vi "Read Analogue.vi"(8 "error in (no error)":errorcluster, 11 "Keysight 6700C in":refnum<class "Keysight 6700C.lvclass">) -> (0 "error out":errorcluster, 2 "Waveforms":waveform(dbl)[](array[waveform]), 3 "Keysight 6700C out":refnum<class "Keysight 6700C.lvclass">)   [LabVIEW 2025, in "Power Supply.lvlib" / "Keysight 6700C.lvclass"]
uses:
  Keysight 6700C.lvclass
  Keysight 6700C.lvclass/Keysight 6700C.ctl
  <instrlib>/Agilent N6700 Series/Agilent N6700 Series.lvlib
  <vilib>/Analysis/NI_AALBase.lvlib
  <vilib>/Analysis/baseanly.llb/Mean (DBL).vi
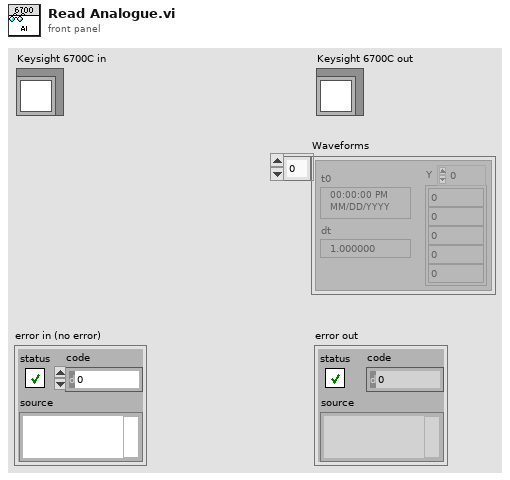
[diagram p1: front panel]
types:
  T1 = typedef "Abstract Engine.lvlibp/Abstract Instrument.lvclass/Channel.ctl" = cluster{"Alias":string, "DataType":enum16{"Anaolg Input", "Waveform"}, "Unit":enum16{"---", "V", "A", "Ohm", "Hz", "uF", "degC", "deg"}, "Upper limit":dbl, "Lower limit":dbl, "Measurement":variant}
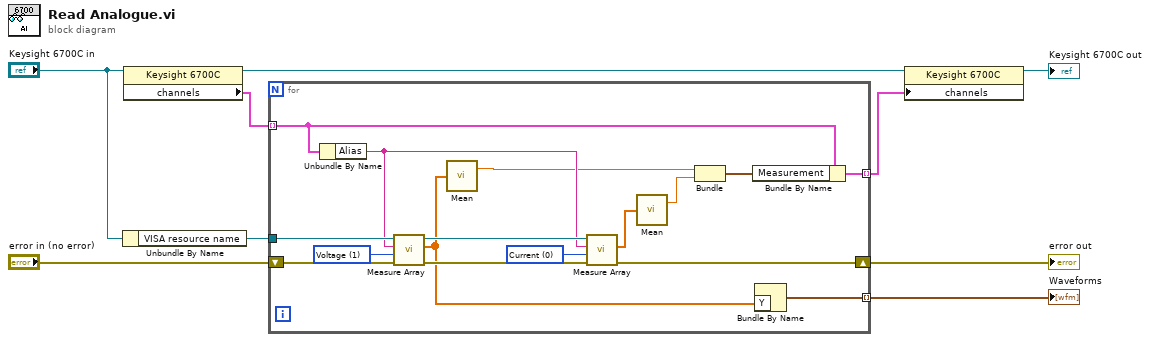
[diagram p0: block diagram]
diagram:
  n1 = Unbundle By Name("Keysight 6700C in") -> ("VISA resource name"=w5:refnum<visa-resource-name>)
  n2 = property class="Keysight 6700C"(reference="Keysight 6700C in") -> (reference out=w4:refnum<class "Keysight 6700C.lvclass">, "channels"=w3:T1[])  [unwired: 1 in, 1 out]
  n3 = for {
    tunnel: w5 -> [w24]
    tunnel: w3 -> [w13] mode=indexing
    shift-right: [w19] -> w6
    shift-left: "error in (no error)" -> [w25]
    tunnel: [w16] -> w2 mode=indexing
    tunnel: [w10] -> w1 mode=indexing
    w21 = 0 items=["Current", "Voltage", "Power"] ("Measurement Type (1: Voltage)")
    w23 = 1 items=["Current", "Voltage", "Power"] ("Measurement Type (1: Voltage)")
    n4 = Unbundle By Name(w13) -> ("Alias"=w15:string)
    n5 = call <instrlib>:"Measure Array.vi"("error in (no error)"=w25, "Measurement Type (1: Voltage)"=w23, "Channel Name (1)"=w15, "VISA resource name"=w24) -> ("error out"=w22:errorcluster, "Measurement Array"=w11:dbl[], "VISA resource name out"=w20:refnum<visa-resource-name>)  [unwired: 4 in, 1 out]
    n6 = call-poly <vilib>:"Mean.vi"("X"=w11) -> ("mean"=w12:dbl)  [unwired: 1 out]
    n7 = call <instrlib>:"Measure Array.vi"("error in (no error)"=w22, "Measurement Type (1: Voltage)"=w21, "Channel Name (1)"=w15, "VISA resource name"=w20) -> ("error out"=w19:errorcluster, "Measurement Array"=w18:dbl[])  [unwired: 4 in, 2 out]
    n8 = call-poly <vilib>:"Mean.vi"("X"=w18) -> ("mean"=w14:dbl)  [unwired: 1 out]
    n9 = Bundle("mean"=w12, "mean"=w14) -> (w17:cluster{"mean":dbl, "mean":dbl})  [unwired: 1 in]
    n10 = Bundle By Name(cluster=w13, "Measurement"=w17) -> (w16:T1)
    n11 = Bundle By Name("Y"=w11) -> (w10:waveform(dbl))  [unwired: 1 in]
  }
  "error out" <- w6
  "Waveforms" <- w1
  n12 = property class="Keysight 6700C"(reference=w4, "channels"=w2) -> (reference out=→"Keysight 6700C out":refnum<class "Keysight 6700C.lvclass">)  [unwired: 1 in, 1 out]
